vi "Do Save VI.vi"(8 "error in (no error)":errorcluster, 10 "save_vi Argument":T3, 11 "Data Cluster in":T1) -> (0 "error out":errorcluster, 2 "VI Path":path, 3 "Data Cluster out":T1)   [LabVIEW 2025, in "Scripting Server.lvlib"]
uses:
  Scripting Server.lvlib
  Module Data--cluster.ctl
  Config Data.ctl
  save_vi Argument--cluster.ctl
  save_vi (Reply Payload)--cluster.ctl
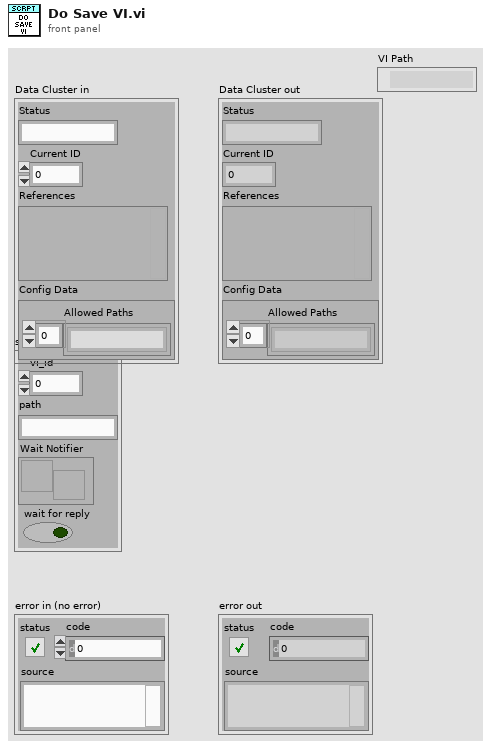
[diagram p1: front panel]
types:
  T1 = typedef "Scripting Server.lvlib/Module Data--cluster.ctl" = cluster{"Status":string, "Current ID":i32, "References":variant, "Config Data":T2}
  T2 = typedef "Scripting Server.lvlib/Config Data.ctl" = cluster{"Allowed Paths":string[]}
  T3 = typedef "Scripting Server.lvlib/save_vi Argument--cluster.ctl" = cluster{"vi_id":i32, "path":string, "Wait Notifier":refnum<notifier>, "wait for reply":bool}
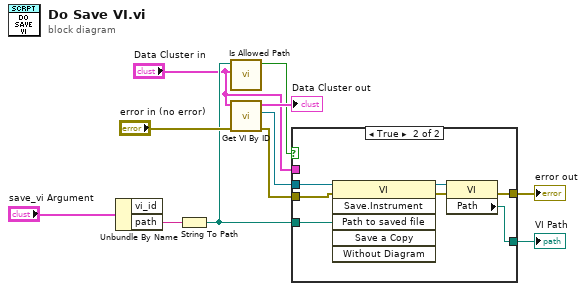
[diagram p0: block diagram]
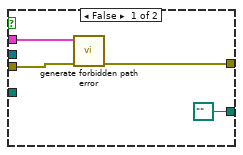
[diagram p2: hidden frame]
diagram:
  n1 = Unbundle By Name("save_vi Argument") -> ("path"=w6:string)  [unwired: 1 out]
  n2 = String To Path(string=w6) -> (path=w3:path)
  n3 = call "Is Allowed Path.vi"("Data Cluster in"="Data Cluster in", "Path"=w3) -> ("Boolean"=w2:bool)  [unwired: 9 in]
  n4 = call "Get VI By ID.vi"("error in (no error)"="error in (no error)", "Data Cluster in"="Data Cluster in") -> ("error out"=w9:errorcluster, "VI Reference"=w7:refnum<vi>, "Data Cluster out"=→"Data Cluster out":T1)  [unwired: 7 in]
  n5 = case shown="True" w2 {
    tunnel: w9 -> [w15 w22]
    tunnel: w7 -> [_ w20]
    tunnel: [w13 w19] -> w5
    tunnel: [path "" ("Path") w17] -> w4
    tunnel: w3 -> [_ w16]
    tunnel: "Data Cluster in" -> [w12 _]
    frame False {
      n6 = call "generate forbidden path error.vi"("error in (no error)"=w15, "Data Cluster in"=w12) -> ("error out"=w13:errorcluster)  [unwired: 9 in]
    }
    frame True {
      n7 = invoke class="VI" method="Save.Instrument"(reference=w20, error in=w22, "Path to saved file"=w16) -> (reference out=w18:refnum<vi>, error out=w21:errorcluster)  [unwired: 3 in, 4 out]
      n8 = property class="VI"(reference=w18, error in=w21) -> (error out=w19:errorcluster, "Path"=w17:path)  [unwired: 1 out]
    }
  }
  "error out" <- w5
  "VI Path" <- w4
